vi "openbci_enable_channels.vi"(8 "error in (no error)":errorcluster, 9 "channel (All channels)":T3, 10 "on? (T)":bool=TRUE, 11 "OBCI dev in":T1={"COM port"="", "n_ch (8)"=enum."8 Channels", "delay_tx"=50}) -> (0 "error out":errorcluster, 3 "OBCI dev out":T1={"COM port"="", "n_ch (8)"=enum."8 Channels", "delay_tx"=50})   [LabVIEW 2013]
doc: "Turn on the respective channel (1-16) by enabling it on the ADS1299\nTurn off the respective channel by disabling it on the ADS1299."
uses:
  Control Def/channels_enum.ctl
  Control Def/openbci_device.ctl
  Control Def/channel_count.ctl
  Control Def/string_channel_off.ctl
  Control Def/string_channel_on.ctl
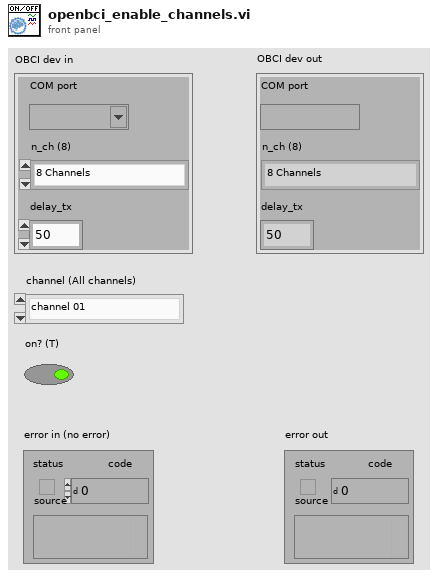
[diagram p1: front panel]
types:
  T1 = typedef "openbci_device.ctl" = cluster{"COM port":refnum<visa-resource-name>, "n_ch (8)":T2, "delay_tx":u32}
  T2 = typedef "channel_count.ctl" = enum16{"8 Channels", "16 Channels"}
  T3 = typedef "channels_enum.ctl" = enum16{"channel 01", "channel 02", "channel 03", "channel 04", "channel 05", "channel 06", "channel 07", "channel 08", "Channel 09", "Channel 10", "Channel 11", "Channel 12", "Channel 13", "Channel 14", "Channel 15", "Channel 16"}
  T4 = typedef "string_channel_on.ctl" = string[]
  T5 = typedef "string_channel_off.ctl" = string[]
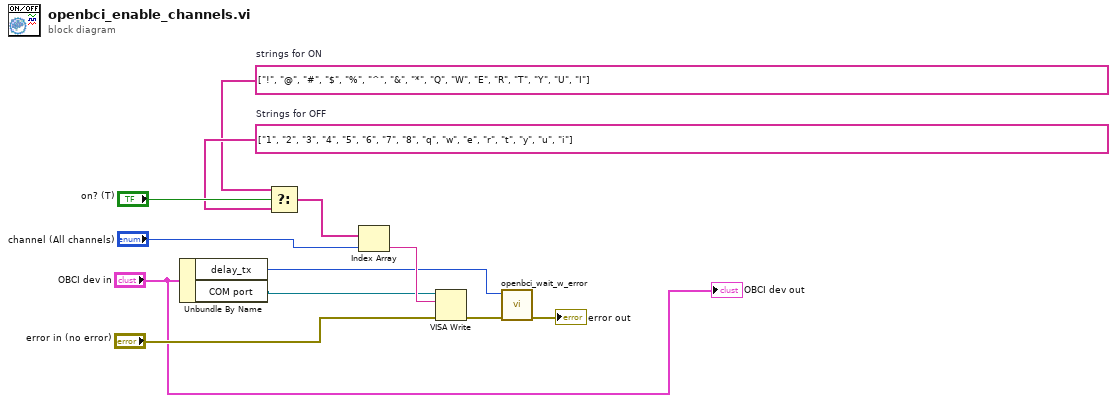
[diagram p0: block diagram]
diagram:
  w9 = T4 ["!", "@", "#", "$", "%", "^", "&", "*", "Q", "W", "E", "R", "T", "Y", "U", "I"]  # strings for ON
  w10 = T5 ["1", "2", "3", "4", "5", "6", "7", "8", "q", "w", "e", "r", "t", "y", "u", "i"]  # Strings for OFF
  n1 = Unbundle By Name("OBCI dev in") -> ("delay_tx"=w2:u32, "COM port"=w5:refnum<visa-resource-name>)
  n2 = Select(t=w9, s="on? (T)", f=w10) -> (s? t:f=w7:T5)
  n3 = Index Array(array=w7, index="channel (All channels)") -> (element=w8:string)
  n4 = VISA Write(VISA resource name=w5, write buffer=w8, error in (no error)="error in (no error)") -> (error out=w4:errorcluster)  [unwired: 2 out]
  n5 = call "openbci_wait_w_error.vi"("error in (no error)"=w4, "milliseconds to wait"=w2) -> ("error out"=→"error out":errorcluster)  [unwired: 9 in]
  "OBCI dev out" <- "OBCI dev in"
